vi "FTW-JSON-Native-HandleErrors.vi"(7 "error in":errorcluster) -> (8 "error out":errorcluster)   [LabVIEW 2015]
uses:
  Error/FTW-ERR-Clear.vi
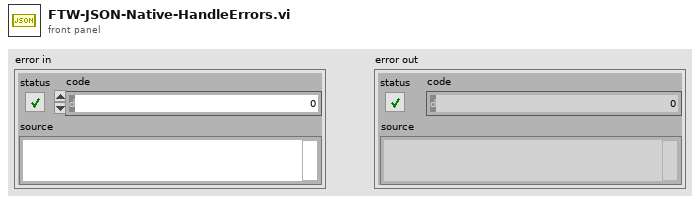
[diagram p1: front panel]
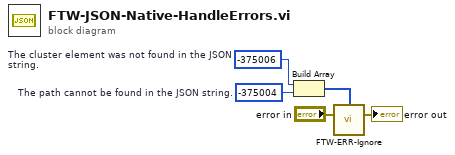
[diagram p0: block diagram]
diagram:
  w1 = -375006  # The cluster element was not found in the JSON string.
  w2 = -375004  # The path cannot be found in the JSON string.
  n1 = Build Array(w1, w2) -> (w3:i32[])
  n2 = call "FTW-ERR-Ignore.vi"("Codes to filter"=w3, "error to filter"="error in") -> ("filtered error"=→"error out":errorcluster)  [unwired: 13 in]
